vi "TestAssetUnary.vi"(0 "Test Input":variant, 1 "Test Output":variant, 3 "error in":errorcluster) -> (7 "Pass?":bool, 10 "error out":errorcluster)   [LabVIEW 2019]
uses:
  <vilib>/Utility/Data Type/NI_Data Type.lvlib
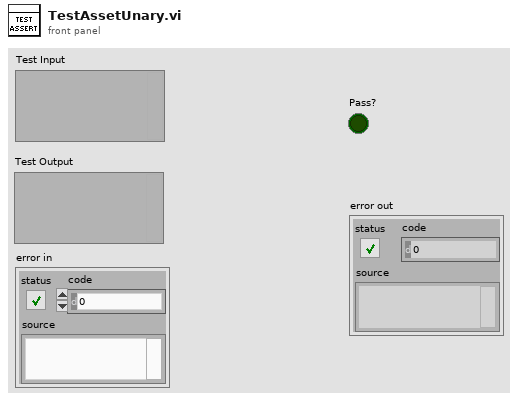
[diagram p1: front panel]
types:
  T1 = typedef "NI_Data Type.lvlib/Data Type.ctl" = enum8{"Invalid Type", "Void", "I8", "I16", "I32", "I64", "U8", "U16", "U32", "U64", "Single Float", "Double Float", "Extended Float", "Single Complex", "Double Complex", "Extended Complex", "Enum U8", "Enum U16", "Enum U32", "Enum U64", "Single Float With Unit", "Double Float With Unit", "Extended Float With Unit", "Single Complex with Unit", "Double Complex with Unit", "Extended Complex with Unit", "Boolean", "String", "Path", "Picture", "Tag", "Array", "Cluster", "Variant", "LV Variant", "Waveform", "Timestamp", "Digital Waveform", "Digital Data", "ExpressData", "Refnum", "External Data", "VI", "Poly VI", "LabVIEW Class Instance", "Fixed Point", "Set Collection", "Map Collection"}
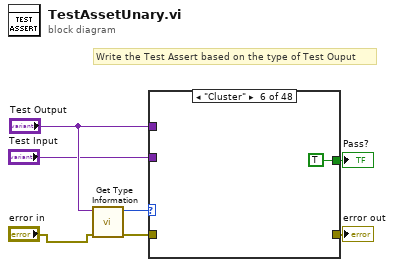
[diagram p0: block diagram]
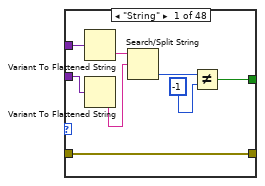
[diagram p2: hidden frame]
diagram:
  # "Write the Test Assert based on the type of Test Ouput"
  n1 = call <vilib>:"Get Type Information.vi"("error in (no error)"="error in", "variant"="Test Output") -> ("error out"=w5:errorcluster, "type"=w7:T1)  [unwired: 5 in, 3 out]
  n2 = case shown="\"Cluster\"" w7 {
    tunnel: w5 -> [w14 _ _ _ _ _ _ _ _ _ _ _ _ _ _ _ _ _ _ _ _ _ _ _ _ _ _ _ _ _ _ _ _ _ _ _ _ _ _ _ _ _ _ _ _ _ _ w19]
    tunnel: "Test Output" -> [w15 _ _ _ _ _ _ _ _ _ _ _ _ _ _ _ _ _ _ _ _ _ _ _ _ _ _ _ _ _ _ _ _ _ _ _ _ _ _ _ _ _ _ _ _ _ _ _]
    tunnel: [w14 _ _ _ _ _ _ _ _ _ _ _ _ _ _ _ _ _ _ _ _ _ _ _ _ _ _ _ _ _ _ _ _ _ _ _ _ _ _ _ _ _ _ _ _ _ _ w18] -> w3
    tunnel: "Test Input" -> [w13 _ _ _ _ _ _ _ _ _ _ _ _ _ _ _ _ _ _ _ _ _ _ _ _ _ _ _ _ _ _ _ _ _ _ _ _ _ _ _ _ _ _ _ _ _ _ _]
    tunnel: [w8 _ _ _ _ TRUE _ _ _ _ _ _ _ _ _ _ _ _ _ _ _ _ _ _ _ _ _ _ _ _ _ _ _ _ _ _ _ _ _ _ _ _ _ _ _ _ _ FALSE] -> w1
    frame "String" {
      n3 = Variant To Flattened String(Variant=w15) -> (data string=w12:string)  [unwired: 1 out]
      n4 = Variant To Flattened String(Variant=w13) -> (data string=w11:string)  [unwired: 1 out]
      n5 = Search/Split String(string=w12, search string/char (-)=w11) -> (offset of match=w10:i32)  [unwired: 1 in, 2 out]
      n6 = Not Equal?(x=w10, y=-1) -> (x != y?=w8:bool)
    }
    frame "Path" {
    }
    frame "Picture" {
    }
    frame "Tag" {
    }
    frame "Array" {
    }
    frame "Cluster" {
    }
    frame "Variant" {
    }
    frame "LV Variant" {
    }
    frame "Waveform" {
    }
    frame "Timestamp" {
    }
    frame "Digital Waveform" {
    }
    frame "Digital Data" {
    }
    frame "ExpressData" {
    }
    frame "Refnum" {
    }
    frame "External Data" {
    }
    frame "VI" {
    }
    frame "Poly VI" {
    }
    frame "LabVIEW Class Instance" {
    }
    frame "Fixed Point" {
    }
    frame "Set Collection" {
    }
    frame "Map Collection" {
    }
    frame "Boolean" {
    }
    frame "Extended Complex with Unit" {
    }
    frame "Double Complex with Unit" {
    }
    frame "Single Complex with Unit" {
    }
    frame "Extended Float With Unit" {
    }
    frame "Double Float With Unit" {
    }
    frame "Single Float With Unit" {
    }
    frame "Enum U64" {
    }
    frame "Enum U32" {
    }
    frame "Enum U16" {
    }
    frame "Enum U8" {
    }
    frame "Extended Complex" {
    }
    frame "Double Complex" {
    }
    frame "Single Complex" {
    }
    frame "Extended Float" {
    }
    frame "Double Float" {
    }
    frame "Single Float" {
    }
    frame "U64" {
    }
    frame "U32" {
    }
    frame "U16" {
    }
    frame "U8" {
    }
    frame "I64" {
    }
    frame "I32" {
    }
    frame "I16" {
    }
    frame "I8" {
    }
    frame "Void" {
    }
    frame "Invalid Type" {
      n7 = Merge Errors(errorcluster {"status"=FALSE, "code"=-1, "source"="Invalid Test output type "} ("error constant"), w19) -> (w18:errorcluster)
    }
  }
  "Pass?" <- w1
  "error out" <- w3
